vi "Write Interface_type.vi"(8 "error in (no error)":errorcluster, 10 "Interface_type":T1="DALI", 11 "_Driver_interaction in":refnum<class "_Driver_interaction.lvclass">) -> (0 "error out":errorcluster, 3 "_Driver_interaction out":refnum<class "_Driver_interaction.lvclass">)   [LabVIEW 2014, in "Driver_interaction.lvlib" / "_Driver_interaction.lvclass"]
uses:
  _Driver_interaction.lvclass
  Controls/Interface_type.ctl
  _Driver_interaction.lvclass/_Driver_interaction.ctl
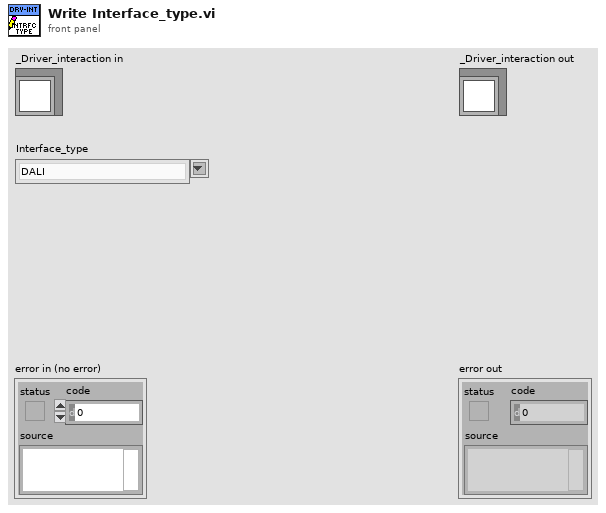
[diagram p1: front panel]
types:
  T1 = typedef "Driver_interaction.lvlib/_Driver_interaction.lvclass/Interface_type.ctl" = string
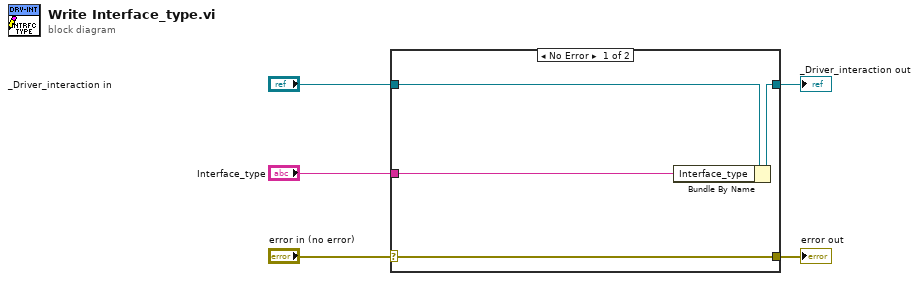
[diagram p0: block diagram]
diagram:
  n1 = case shown="No Error" "error in (no error)" {
    selector: "error in (no error)" -> [w9 w10]
    tunnel: [w9 w10] -> w4
    tunnel: [w7 w11] -> w2
    tunnel: "_Driver_interaction in" -> [w8 w11]
    tunnel: "Interface_type" -> [w6 _]
    frame No Error {
      n2 = Bundle By Name(cluster=w8, "Interface_type"=w6) -> (w7:refnum<class "_Driver_interaction.lvclass">)
    }
    frame Error {
    }
  }
  "error out" <- w4
  "_Driver_interaction out" <- w2
